vi "拉取依赖文件并更新.vi"(8 "error in (no error)":errorcluster, 11 "远端地址":string="/updatefiles/OneStation/V4/一体化微型水质监测站.zip") -> (0 "error out":errorcluster)   [LabVIEW 2016, in "数据传输系统-06.lvlib" / "update.lvlib" / "http client.lvclass"]
uses:
  http client.lvclass
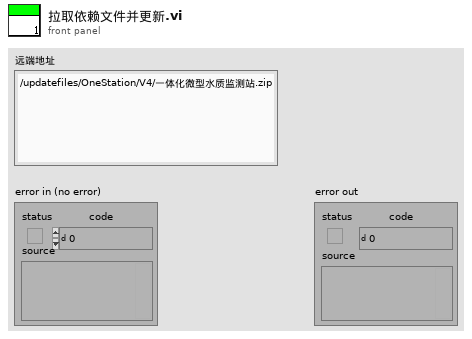
[diagram p1: front panel]
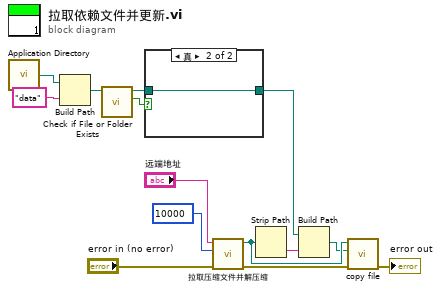
[diagram p0: block diagram]
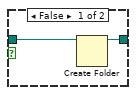
[diagram p2: hidden frame]
diagram:
  n1 = call <vilib>:"Application Directory.vi"() -> ("Application Directory"=w12:path)
  n2 = Build Path(base path=w12, name or relative path="data" ("名称或相对路径")) -> (appended path=w4:path)
  n3 = call <vilib>:"Check if File or Folder Exists.vi"("path"=w4) -> ("file or folder exists?"=w2:bool, "dup path"=w3:path)  [unwired: 8 in, 1 out]
  n4 = case shown="真" w2 {
    tunnel: w3 -> [w16 w17]
    tunnel: [w15 w17] -> w5
    frame False {
      n5 = Create Folder(path (use dialog)=w16) -> (created path=w15:path)  [unwired: 2 in, 2 out]
    }
    frame True {
    }
  }
  n6 = call "拉取压缩文件并解压缩.vi"("error in (no error)"="error in (no error)", "timeout (10000)"=10000, "远端地址"="远端地址") -> ("error out"=w14:errorcluster, "文件路径"=w10:path)  [unwired: 7 in]
  n7 = Strip Path(path=w10) -> (name=w9:string)  [unwired: 1 out]
  n8 = Build Path(base path=w5, name or relative path=w9) -> (appended path=w8:path)
  n9 = call "copy file.vi"("error in (no error)"=w14, "目标路径（使用对话框）"=w8, "源路径"=w10) -> ("error out"=→"error out":errorcluster)  [unwired: 8 in]
